vi "Example gRPC Client Call.vi"() -> ()   [LabVIEW 2016]
uses:
  D:/GitHub/LabVIEW/gRPC/labview-grpc-client-using-CSharp/Client/C# Client/bin/release/net461/ExampleCSharpClient.dll
  C# Client/bin/release/net461/ExampleCSharpClient.dll
  D:/GitHub/LabVIEW/gRPC/labview-grpc-client-using-CSharp/Client/C# Client/bin/release/net461/Grpc.Core.Api.dll
  C# Client/bin/release/net461/Grpc.Core.Api.dll
  D:/GitHub/LabVIEW/gRPC/labview-grpc-client-using-CSharp/Client/C# Client/bin/release/net461/Grpc.Core.dll
  C# Client/bin/release/net461/Grpc.Core.dll
panel:
  out "Message (Uptime in sec)":string
  out "error out":errorcluster
  out "Status":i32
  in  "Query":string="Uptime"
  in  "target":string="localhost:50051"
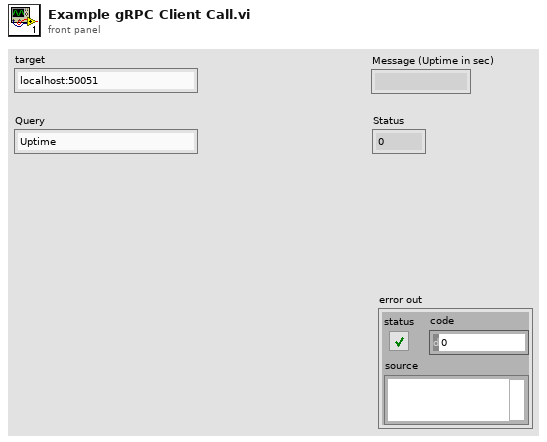
[diagram p1: front panel]
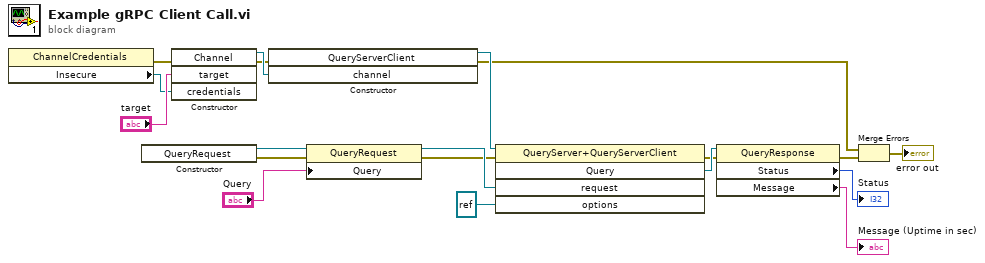
[diagram p0: block diagram]
diagram:
  n1 = property class="ChannelCredentials"() -> (error out=w4:errorcluster, "Insecure"=w3:refnum<k24>)  [unwired: 2 in, 1 out]
  n2 = constructor class="QueryRequest"() -> (reference out=w19:refnum<k24>, error out=w18:errorcluster)  [unwired: 3 in, 1 out]
  n3 = constructor class="Channel"(error in=w4, "target"="target", "credentials"=w3) -> (reference out=w16:refnum<k24>, error out=w11:errorcluster)  [unwired: 2 in, 3 out]
  n4 = constructor class="QueryServer+QueryServerClient"(error in=w11, "channel"=w16) -> (reference out=w15:refnum<k24>, error out=w8:errorcluster)  [unwired: 2 in, 2 out]
  n5 = property class="QueryRequest"(reference=w19, error in=w18, "Query"="Query") -> (reference out=w14:refnum<k24>, error out=w10:errorcluster)
  n6 = invoke class="QueryServer+QueryServerClient" method="Query"(reference=w15, error in=w10, "request"=w14, "options"=refnum<k24> refnum) -> (error out=w9:errorcluster, "Query"=w13:refnum<k24>)  [unwired: 1 in, 3 out]
  n7 = property class="QueryResponse"(reference=w13, error in=w9) -> (error out=w7:errorcluster, "Status"=→"Status":i32, "Message"=→"Message (Uptime in sec)":string)  [unwired: 1 out]
  n8 = Merge Errors(w8, w7) -> (→"error out":errorcluster)
